vi "TDMS Copy File.vi"(8 "error in":errorcluster, 10 "tdms dest in":refnum<k34>, 11 "tdms source in":refnum<k34>) -> (0 "error out":errorcluster, 2 "tdms dest out":refnum<k34>, 3 "tdms source out":refnum<k34>)   [LabVIEW 2011]
doc: "Copies all the channels and properties from the source file to the destination file."
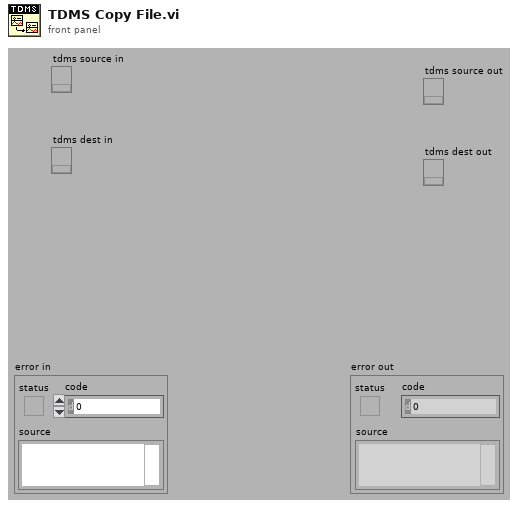
[diagram p1: front panel]
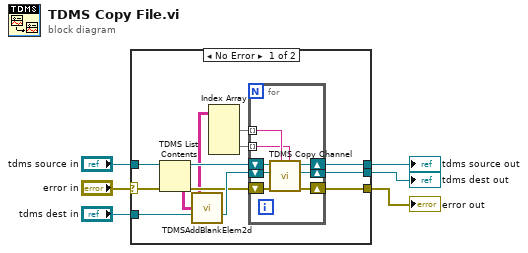
[diagram p0: block diagram]
diagram:
  n1 = case shown="No Error" "error in" {
    selector: "error in" -> [w8 w29]
    tunnel: "tdms dest in" -> [w18 w27]
    tunnel: "tdms source in" -> [w17 w28]
    tunnel: [w14 w28] -> w4
    tunnel: [w13 w27] -> w3
    tunnel: [w9 w29] -> w2
    frame No Error {
      n2 = TDMS List Contents(4:w8, 7:w17) -> (0:w16:errorcluster, 1:w7:string[][], 3:w15:refnum<k34>)  [unwired: 2 out]
      n3 = call <vilib>:"TDMSAddBlankElem2d.vi"("input 2d string array"=w7) -> ("output 2d string array with the first column blank"=w12:string[][])
      n4 = Index Array(array=w12) -> (element #1=w11:string[], element #2=w10:string[])  [unwired: 4 in]
      n5 = for {
        shift-right: [w25] -> w9
        shift-left: w16 -> [w22]
        shift-right: [w24] -> w13
        shift-left: w18 -> [w26]
        shift-right: [w23] -> w14
        shift-left: w15 -> [w21]
        tunnel: w11 -> [w20] mode=indexing
        tunnel: w10 -> [w19] mode=indexing
        n6 = call "TDMS Copy Channel.vi"("channel name"=w19, "group name"=w20, "error in"=w22, "tdms dest in"=w26, "tdms source in"=w21) -> ("error out"=w25:errorcluster, "tdms dest out"=w24:refnum<k34>, "tdms source out"=w23:refnum<k34>)  [unwired: 4 out]
      }
    }
    frame Error {
    }
  }
  "tdms source out" <- w4
  "tdms dest out" <- w3
  "error out" <- w2
